vi "Obtain Request Events.vi"(8 "error in (no error)":errorcluster, 10 "Create New?":bool) -> (0 "error out":errorcluster, 2 "Data Logger v2 Request Events":T1)   [LabVIEW 2025, in "Data Logger v2.lvlib"]
doc: "This VI Obtains/Creates the Requests events that will be used for other modules to communicate with the module that owns this VI. These Requests events will be accessed only via Public API methods for this module.\n\n<b>NOTE</b>: The contents of this VI are automatically generated and modified by the <b>Tools > Delacor > DQMH</b> utilities. Consider using those utilities instead of making your own modifications to this VI.\n_____\nBased on Delacor QMH Project Template 3.1.0.34."
uses:
  Data Logger v2.lvlib
  Request Events--cluster.ctl
  Stop Argument--cluster.ctl
  Show Panel Argument--cluster.ctl
  Hide Panel Argument--cluster.ctl
  Get Module Execution Status Argument--cluster.ctl
  Show Diagram Argument--cluster.ctl
  Change Panel Argument--cluster.ctl
  <vilib>/MGI/Panel Manager/Panel/Panel/Panel.lvclass
  Create New TDMS Log File Argument--cluster.ctl
  Write 2D Array to TDMS Log File Argument--cluster.ctl
  Write TDMS 2D Array Parameters--cluster.ctl
  Close TDMS File Argument--cluster.ctl
  Write TDMS 2D String Array Argument--cluster.ctl
  Write TDMS 2D String Array Parameters--cluster.ctl
  Set Root Folder Path Argument--cluster.ctl
  Create New TDMS Log File (Relative Path) Argument--cluster.ctl
  Set Properties Argument--cluster.ctl
panel:
  # "NOTE: The contents of this VI are automatically generated and modified by the Tools > Delacor > DQMH utilities. Consider using those utilities instead of making your own modifications to this VI."
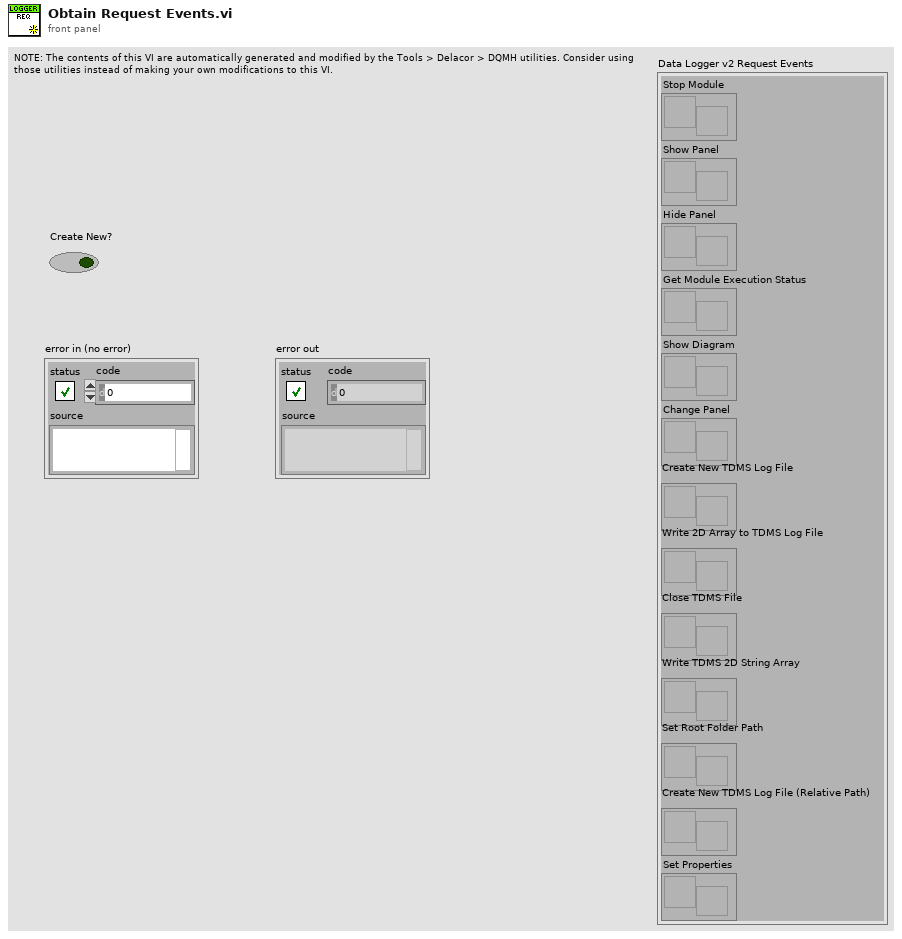
[diagram p1: front panel]
types:
  T1 = typedef "Data Logger v2.lvlib/Request Events--cluster.ctl" = cluster{"Stop Module":refnum<user-event>, "Show Panel":refnum<user-event>, "Hide Panel":refnum<user-event>, "Get Module Execution Status":refnum<user-event>, "Show Diagram":refnum<user-event>, "Change Panel":refnum<user-event>, "Create New TDMS Log File":refnum<user-event>, "Write 2D Array to TDMS Log File":refnum<user-event>, "Close TDMS File":refnum<user-event>, "Write TDMS 2D String Array":refnum<user-event>, "Set Root Folder Path":refnum<user-event>, "Create New TDMS Log File (Relative Path)":refnum<user-event>, "Set Properties":refnum<user-event>}
  T2 = typedef "Data Logger v2.lvlib/Set Properties Argument--cluster.ctl" = cluster{"Property names":string[], "Property values":variant[], "Group name":string, "Channel name":string}
  T3 = typedef "Data Logger v2.lvlib/Create New TDMS Log File (Relative Path) Argument--cluster.ctl" = cluster{"Filename":string}
  T4 = typedef "Data Logger v2.lvlib/Set Root Folder Path Argument--cluster.ctl" = cluster{"Root Folder Path":path}
  T5 = typedef "Data Logger v2.lvlib/Write TDMS 2D String Array Argument--cluster.ctl" = cluster{"TDMS Write 2D String Array Parameters":T6}
  T6 = typedef "Data Logger v2.lvlib/Write TDMS 2D String Array Parameters--cluster.ctl" = cluster{"Group":string, "Channel Names":string[], "Data":string[][]}
  T7 = typedef "Data Logger v2.lvlib/Close TDMS File Argument--cluster.ctl" = cluster{"Boolean":bool}
  T8 = typedef "Data Logger v2.lvlib/Write 2D Array to TDMS Log File Argument--cluster.ctl" = cluster{"TDMS Write 2D Array Parameters":T9}
  T9 = typedef "Data Logger v2.lvlib/Write TDMS 2D Array Parameters--cluster.ctl" = cluster{"Group":string, "Channel Names":string[], "Data":dbl[][]}
  T10 = typedef "Data Logger v2.lvlib/Create New TDMS Log File Argument--cluster.ctl" = cluster{"File Path (inc. Filename)":path}
  T11 = typedef "Data Logger v2.lvlib/Change Panel Argument--cluster.ctl" = cluster{"New Panel":refnum<class "Panel.lvclass">}
  T12 = typedef "Data Logger v2.lvlib/Hide Panel Argument--cluster.ctl" = cluster{"Hide Panel?":bool}
  T13 = typedef "Data Logger v2.lvlib/Show Panel Argument--cluster.ctl" = cluster{"Show Panel?":bool}
  T14 = typedef "Data Logger v2.lvlib/Show Diagram Argument--cluster.ctl" = cluster{"Debug?":bool}
  T15 = typedef "Data Logger v2.lvlib/Get Module Execution Status Argument--cluster.ctl" = cluster{"Running?":bool}
  T16 = typedef "Data Logger v2.lvlib/Stop Argument--cluster.ctl" = cluster{"Origin":string, "Exit via Stop Module Req?":bool, "Wait for Module to stop?":bool}
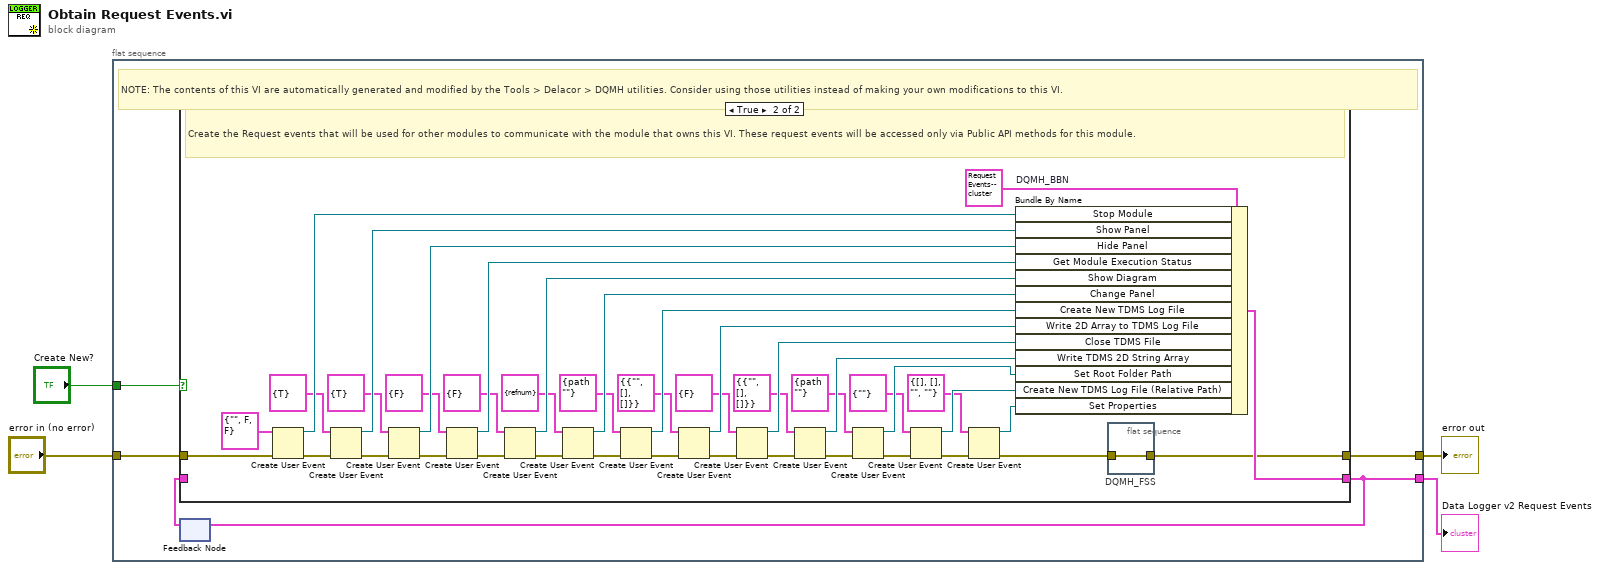
[diagram p0: block diagram]
diagram:
  n1 = flat-sequence {
    tunnel: [w9] -> w4
    tunnel: "error in (no error)" -> [w8]
    tunnel: [w6] -> w2
    tunnel: "Create New?" -> [w5]
    frame #0 {
      # "NOTE: The contents of this VI are automatically generated and modified by the Tools > Delacor > DQMH utilities. Consider using those utilities instead of making your own modifications to this VI."
      n2 = feedback #1() -> (w7:T1)  [unwired: 1 in]
      n3 = case shown="True" w5 {
        tunnel: [w10 w44] -> w9
        tunnel: w8 -> [w10 w54]
        tunnel: [w11 w51] -> w6
        tunnel: w7 -> [w11 _]
        frame False {
          # "Obtain the Request events that were created in a previous call to this VI."
        }
        frame True {
          # "Create the Request events that will be used for other modules to communicate with the module that owns this VI. These request events will be accessed only via Public API methods for this module."
          n4 = Create User Event(user event datatype=T16 {"Origin"="", "Exit via Stop Module Req?"=FALSE, "Wait for Module to stop?"=FALSE} ("Stop Argument"), error in=w54) -> (user event=w52:refnum<user-event>, error out=w49:errorcluster)
          n5 = Create User Event(user event datatype=T13 {"Show Panel?"=TRUE} ("Show Panel Argument"), error in=w49) -> (user event=w48:refnum<user-event>, error out=w47:errorcluster)
          n6 = Create User Event(user event datatype=T12 {"Hide Panel?"=TRUE} ("Hide Panel Argument"), error in=w47) -> (user event=w46:refnum<user-event>, error out=w45:errorcluster)
          n7 = Create User Event(user event datatype=T15 {"Running?"=FALSE} ("Get Module Execution Status Argument"), error in=w45) -> (user event=w42:refnum<user-event>, error out=w43:errorcluster)
          n8 = Create User Event(user event datatype=T14 {"Debug?"=FALSE} ("Show Diagram Argument"), error in=w43) -> (user event=w39:refnum<user-event>, error out=w40:errorcluster)
          n9 = Create User Event(user event datatype=T11 {"New Panel"=refnum} ("Change Panel Argument"), error in=w40) -> (user event=w34:refnum<user-event>, error out=w35:errorcluster)
          n10 = Create User Event(user event datatype=T10 {"File Path (inc. Filename)"=path ""} ("Create New TDMS Log File Argument"), error in=w35) -> (user event=w31:refnum<user-event>, error out=w32:errorcluster)
          n11 = Create User Event(user event datatype=T8 {"TDMS Write 2D Array Parameters"={"Group"="", "Channel Names"=[], "Data"=[]}} ("Write 2D Array to TDMS Log File Argument"), error in=w32) -> (user event=w28:refnum<user-event>, error out=w29:errorcluster)
          n12 = Create User Event(user event datatype=T7 {"Boolean"=FALSE} ("Close TDMS File Argument"), error in=w29) -> (user event=w25:refnum<user-event>, error out=w26:errorcluster)
          n13 = Create User Event(user event datatype=T5 {"TDMS Write 2D String Array Parameters"={"Group"="", "Channel Names"=[], "Data"=[]}} ("Write TDMS 2D String Array Argument"), error in=w26) -> (user event=w22:refnum<user-event>, error out=w23:errorcluster)
          n14 = Create User Event(user event datatype=T4 {"Root Folder Path"=path ""} ("Set Root Folder Path Argument"), error in=w23) -> (user event=w19:refnum<user-event>, error out=w20:errorcluster)
          n15 = Create User Event(user event datatype=T3 {"Filename"=""} ("Create New TDMS Log File (Relative Path) Argument"), error in=w20) -> (user event=w16:refnum<user-event>, error out=w17:errorcluster)
          n16 = Create User Event(user event datatype=T2 {"Property names"=[], "Property values"=[], "Group name"="", "Channel name"=""} ("Set Properties Argument"), error in=w17) -> (user event=w13:refnum<user-event>, error out=w14:errorcluster)
          n17 = Bundle By Name "DQMH_BBN"(cluster=T1 {"Stop Module"=refnum, "Show Panel"=refnum, "Hide Panel"=refnum, "Get Module Execution Status"=refnum, "Show Diagram"=refnum, "Change Panel"=refnum, "Create New TDMS Log File"=refnum, "Write 2D Array to TDMS Log File"=refnum, "Close TDMS File"=refnum, "Write TDMS 2D String Array"=refnum, "Set Root Folder Path"=refnum, "Create New TDMS Log File (Relative Path)"=refnum, "Set Properties"=refnum} ("output cluster"), "Stop Module"=w52, "Show Panel"=w48, "Hide Panel"=w46, "Get Module Execution Status"=w42, "Show Diagram"=w39, "Change Panel"=w34, "Create New TDMS Log File"=w31, "Write 2D Array to TDMS Log File"=w28, "Close TDMS File"=w25, "Write TDMS 2D String Array"=w22, "Set Root Folder Path"=w19, "Create New TDMS Log File (Relative Path)"=w16, "Set Properties"=w13) -> (w51:T1)
          n18 = flat-sequence "DQMH_FSS" {
            tunnel: w14 -> [w55]
            tunnel: [w55] -> w44
            frame #0 {
            }
          }
        }
      }
      n19 = feedback-in #1(w6) -> ()
    }
  }
  "Data Logger v2 Request Events" <- w2
  "error out" <- w4
